vi "Send Write System Status Ref.vi"(7 "Message Priority (Normal)":T1=enum."Normal", 8 "error in (no error)":errorcluster, 10 "System Status Ref":refnum<vi>, 11 "Message Enqueuer":refnum<class "Message Enqueuer.lvclass">) -> (0 "error out":errorcluster, 3 "Message Enqueuer out":refnum<class "Message Enqueuer.lvclass">)   [LabVIEW 2014, in "Robot Actor Framework.lvlib" / "System Actor.lvlib" / "Write System Status Ref Msg.lvclass"]
doc: "This VI sends the message to an actor."
uses:
  Write System Status Ref Msg.lvclass
  <vilib>/ActorFramework/Message Enqueuer/Message Enqueuer.lvclass
  <vilib>/ActorFramework/Message Enqueuer/Message Priority.ctl
  System Actor Class/System State.ctl
  Command Actor/Command Actor Class/Command State.ctl
  Command Actor/Command Actor Class/Command States.ctl
  Command Processor Actor/Command Processor Actor Class/Command Processor State.ctl
  Command Processor Actor/Command Processor Actor Class/Command Processor States.ctl
  Write System Status Ref Msg.lvclass/Write System Status Ref Msg.ctl
  <vilib>/ActorFramework/Message Enqueuer/Message Enqueuer.lvclass/Message Enqueuer.ctl
  <vilib>/ActorFramework/Message Priority Queue/Priority Enqueue.vi
  Command Actor/Command Actor Class/Command Actor.lvclass
  System Actor Class/System Actor.lvclass
  Command Processor Actor/Command Processor Actor Class/Command Processor Actor.lvclass
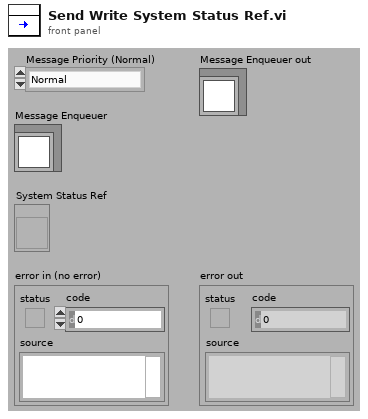
[diagram p1: front panel]
types:
  T1 = typedef "Actor Framework.lvlib/Message Enqueuer.lvclass/Message Priority.ctl" = enum16{"Low", "Normal", "High"}
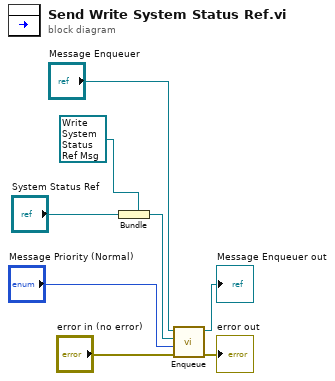
[diagram p0: block diagram]
diagram:
  n1 = Bundle(cluster=refnum<class "Write System Status Ref Msg.lvclass"> refnum ("Object"), "System Status Ref") -> (w4:refnum<class "Write System Status Ref Msg.lvclass">)
  n2 = call <vilib>:"Enqueue.vi"("error in (no error)"="error in (no error)", "Message Priority (Normal)"="Message Priority (Normal)", "Message"=w4, "Message Enqueuer in"="Message Enqueuer") -> ("error out"=→"error out":errorcluster, "Message Enqueuer out"=→"Message Enqueuer out":refnum<class "Message Enqueuer.lvclass">)  [unwired: 6 in]
